vi "Host - Is Download Necessary.vi"(8 "Error In (no error)":errorcluster, 9 "bitfile path in":path, 10 "Target IP Address in":string, 11 "Slave Ref in":refnum<k21>) -> (0 "error out":errorcluster, 1 "bitfile path out":path, 2 "Target IP Address out":string, 3 "Slave Ref out":refnum<k21>, 5 "is download necessary?":bool)   [LabVIEW 2016, in "Scan Engine Custom Device.lvlib"]
uses:
  Scan Engine Custom Device.lvlib
panel:
  out "error IO":errorcluster
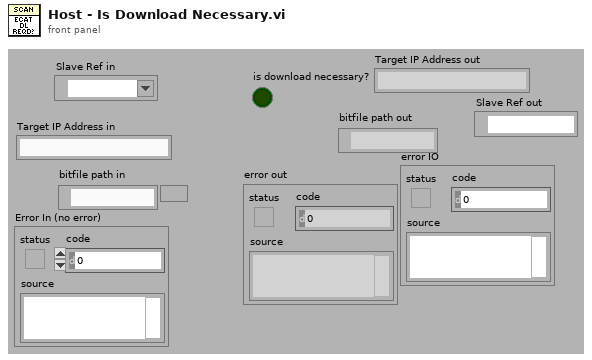
[diagram p1: front panel]
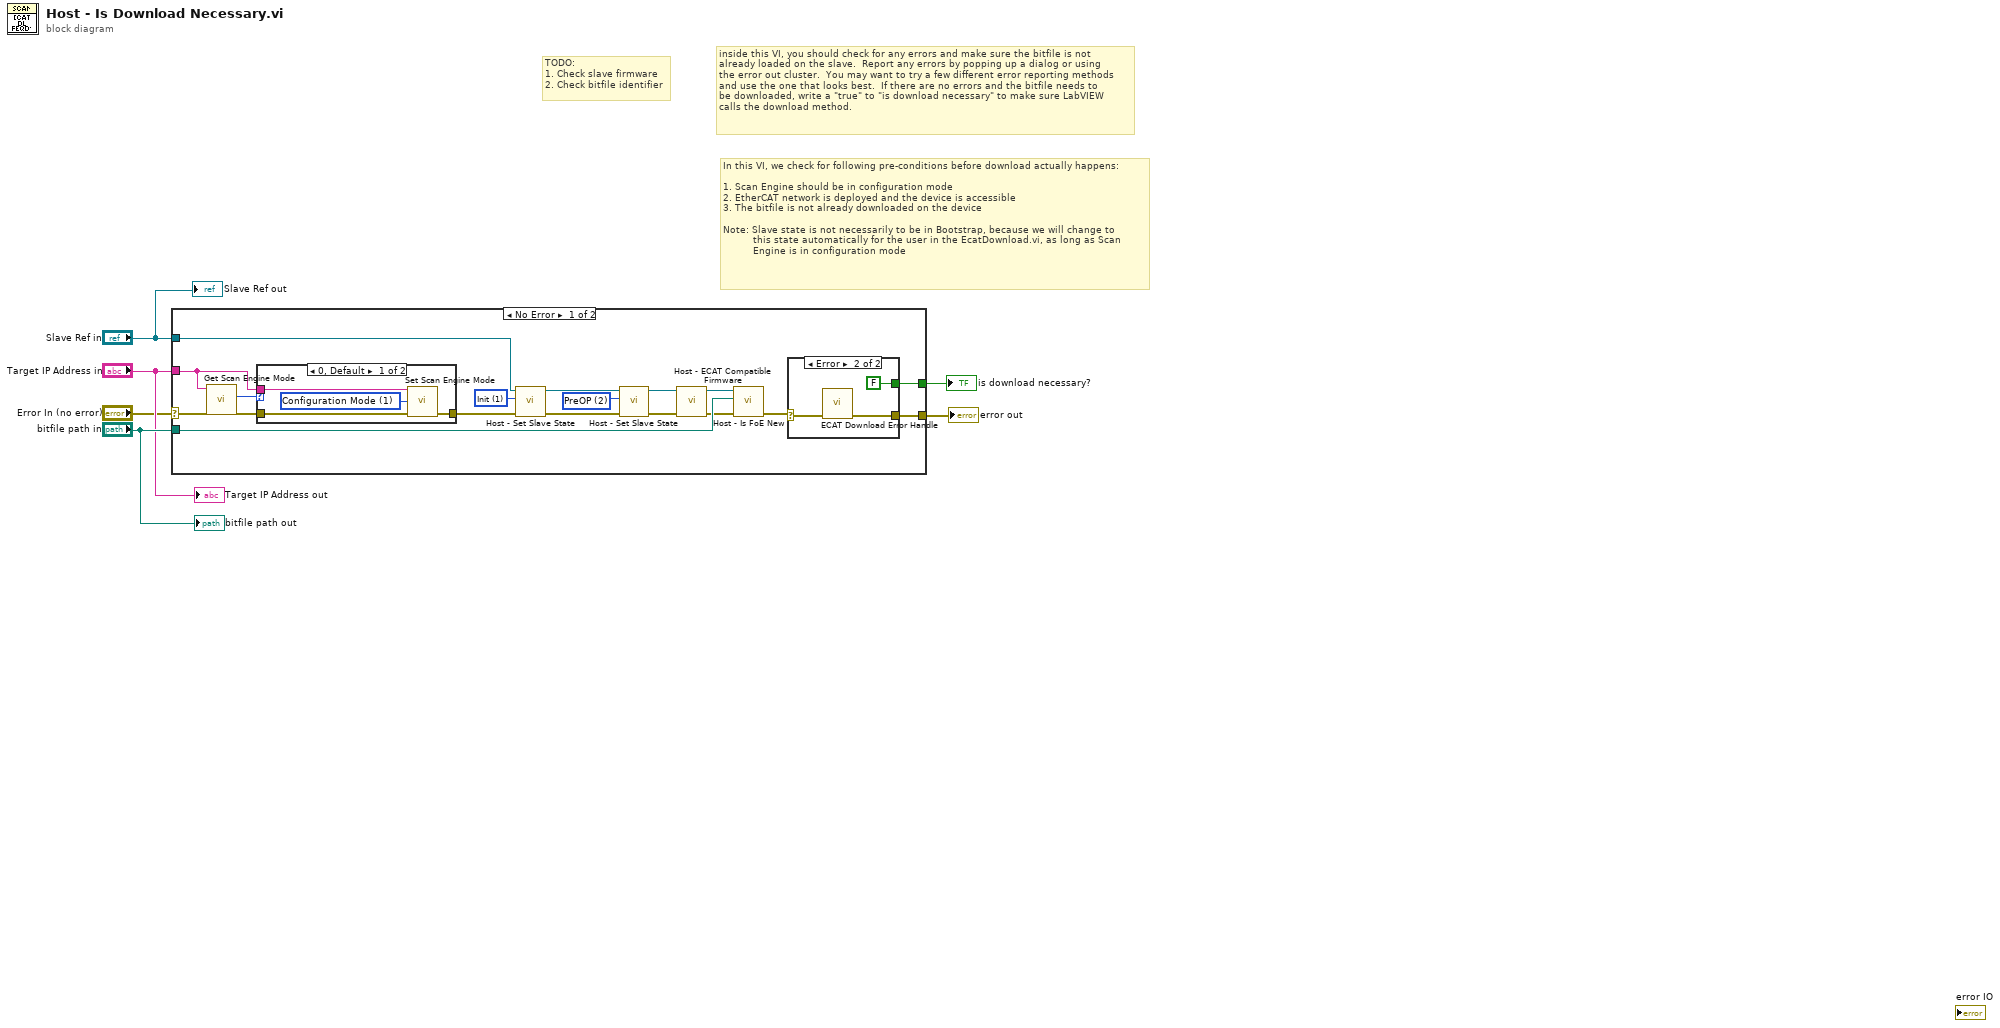
[diagram p0: block diagram]
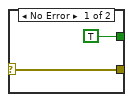
[diagram p3: hidden frame]
diagram:
  # "TODO:\n1. Check slave firmware\n2. Check bitfile identifier"
  # "In this VI, we check for following pre-conditions before download actually happens:\n\n1. Scan Engine should be in configuration mode\n2. EtherCAT network is deployed and the device is accessible\n3. The bitfile is not already downloaded on the device\n\nNote: Slave state is not necessarily to be in Bootstrap, because we will change to\n          this state automatically for the user in the EcatDownload.vi, as long as Scan\n          Engine is in configuration mode"
  # "inside this VI, you should check for any errors and make sure the bitfile is not\nalready loaded on the slave.  Report any errors by popping up a dialog or using \nthe error out cluster.  You may want to try a few different error reporting methods\nand use the one that looks best.  If there are no errors and the bitfile needs to\nbe downloaded, write a \"true\" to \"is download necessary\" to make sure LabVIEW\ncalls the download method."
  n1 = case shown="No Error" "Error In (no error)" {
    selector: "Error In (no error)" -> [w17 w35]
    tunnel: "bitfile path in" -> [w24 _]
    tunnel: [w23 w35] -> w5
    tunnel: [w21 _] -> w4
    tunnel: "Target IP Address in" -> [w16 _]
    tunnel: "Slave Ref in" -> [w20 _]
    frame No Error {
      w13 = u32 2 items=["Init"=1, "PreOP"=2, "BootStrap"=3, "SafeOP"=4, "OP"=8] ("slaveState")
      w14 = u32 1 items=["Init"=1, "PreOP"=2, "BootStrap"=3, "SafeOP"=4, "OP"=8] ("slaveState")
      n2 = call <vilib>:"Get Scan Engine Mode.vi"("error in (no error)"=w17, "target address (localhost)"=w16) -> ("error out"=w19:errorcluster, "mode"=w18:i32)  [unwired: 8 in]
      n3 = case shown="0, Default" w18 {
        tunnel: w16 -> [w27 _]
        tunnel: w19 -> [w26 w29]
        tunnel: [w25 w29] -> w15
        frame 0, Default {
          w28 = 1 items=["Configuration Mode"=1, "Active Mode"=2] ("mode (Active Mode)")
          n4 = call <vilib>:"Set Scan Engine Mode.vi"("target address (localhost)"=w27, "mode (Active Mode)"=w28, "error in (no error)"=w26) -> ("error out"=w25:errorcluster)  [unwired: 12 in]
        }
        frame 1 {
        }
      }
      n5 = call "Host - Set Slave State.vi"("error in (no error)"=w15, "slaveState"=w14, "Slave Ref in"=w20) -> ("error out"=w11:errorcluster, "Slave Ref out"=w12:refnum<k21>)  [unwired: 5 in, 2 out]
      n6 = call "Host - Set Slave State.vi"("error in (no error)"=w11, "slaveState"=w13, "Slave Ref in"=w12) -> ("error out"=w9:errorcluster, "Slave Ref out"=w10:refnum<k21>)  [unwired: 5 in, 2 out]
      n7 = call "Host - ECAT Compatible Firmware.vi"("error in (no error)"=w9, "Slave Ref in"=w10) -> ("error out"=w7:errorcluster, "Slave Ref out"=w8:refnum<k21>)  [unwired: 8 in]
      n8 = call "Host - Is FoE New.vi"("error in (no error)"=w7, "bitfile path in"=w24, "Slave Ref in"=w8) -> ("error out"=w22:errorcluster)  [unwired: 7 in, 1 out]
      n9 = case shown="Error" w22 {
        selector: w22 -> [w31 w33]
        tunnel: [w31 w34] -> w23
        tunnel: [TRUE ("is download necessary") FALSE ("is download necessary")] -> w21
        frame No Error {
        }
        frame Error {
          n10 = call "ECAT Download Error Handle.vi"("error in"=w33) -> ("error out"=w34:errorcluster)  [unwired: 10 in]
        }
      }
    }
    frame Error {
    }
  }
  "is download necessary?" <- w4
  "error out" <- w5
  "Target IP Address out" <- "Target IP Address in"
  "bitfile path out" <- "bitfile path in"
  "Slave Ref out" <- "Slave Ref in"
